vi "UI Set State.vi"(8 "error in (no error)":errorcluster, 10 "State Type":string, 11 "UI Refs":T1) -> (0 "error out":errorcluster, 3 "dup UI Refs":T1)   [LabVIEW 2015]
uses:
  controls/UI Data.ctl
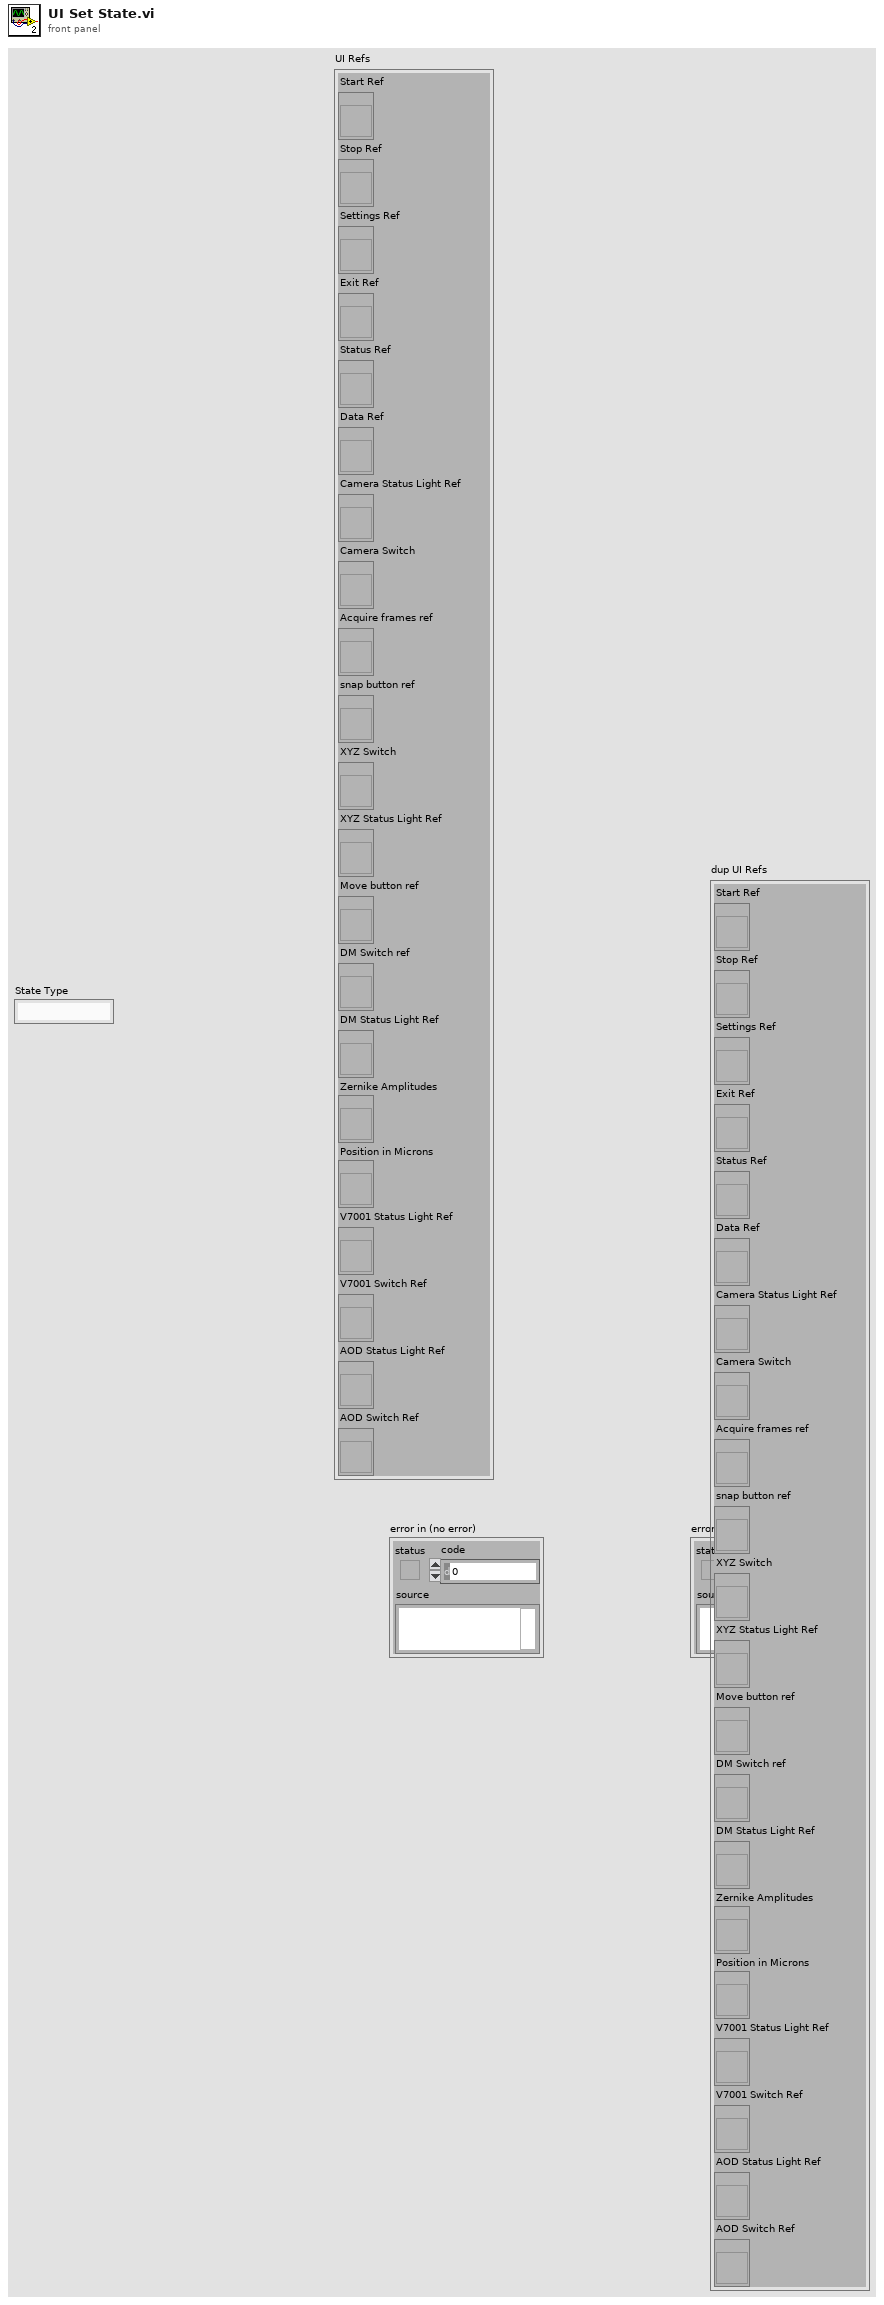
[diagram p1: front panel]
types:
  T1 = typedef "UI Data.ctl" = cluster{"Start Ref":refnum<vi>, "Stop Ref":refnum<vi>, "Settings Ref":refnum<vi>, "Exit Ref":refnum<vi>, "Status Ref":refnum<vi>, "Data Ref":refnum<vi>, "Camera Status Light Ref":refnum<vi>, "Camera Switch":refnum<vi>, "Acquire frames ref":refnum<vi>, "snap button ref":refnum<vi>, "XYZ Switch":refnum<vi>, "XYZ Status Light Ref":refnum<vi>, "Move button ref":refnum<vi>, "DM Switch ref":refnum<vi>, "DM Status Light Ref":refnum<vi>, "Zernike Amplitudes":refnum<vi>, "Position in Microns":refnum<vi>, "V7001 Status Light Ref":refnum<vi>, "V7001 Switch Ref":refnum<vi>, "AOD Status Light Ref":refnum<vi>, "AOD Switch Ref":refnum<vi>}
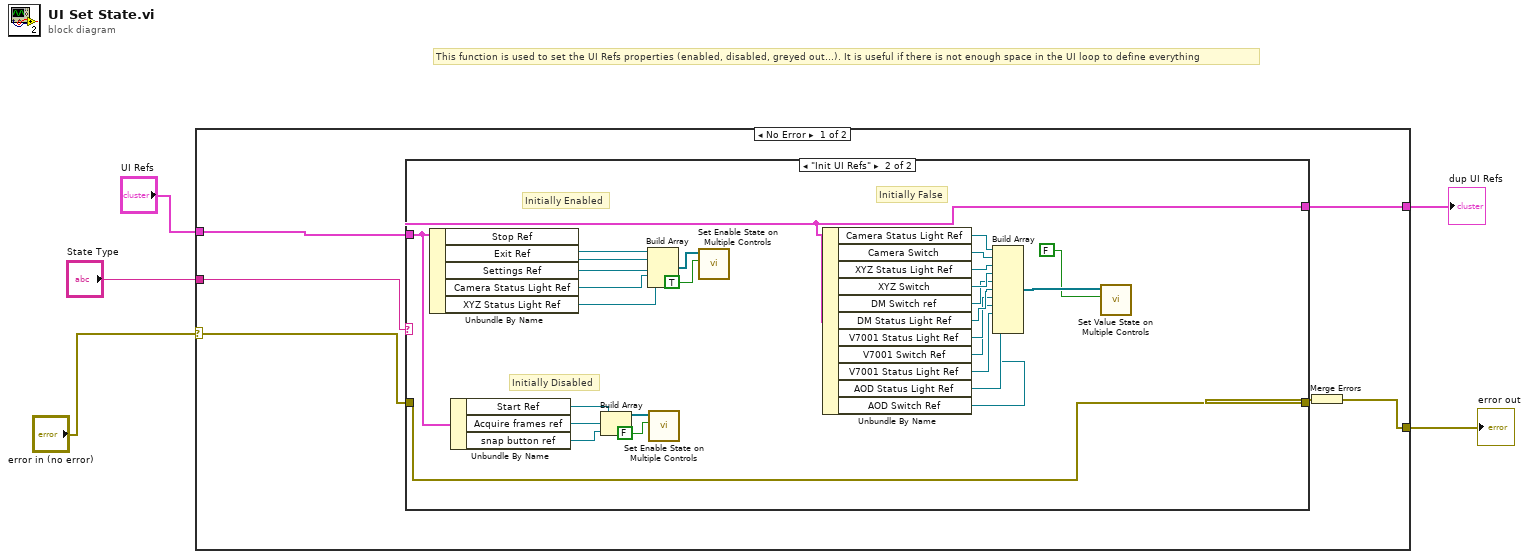
[diagram p0: block diagram]
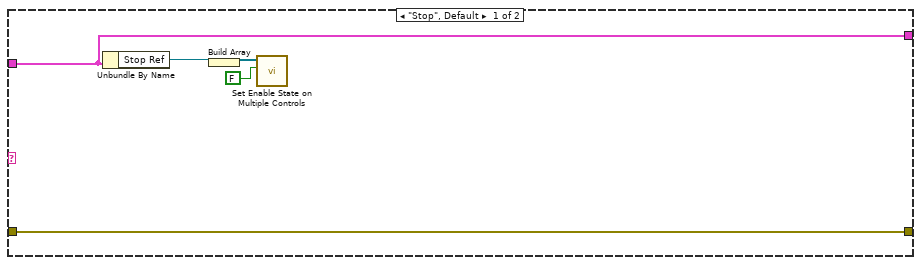
[diagram p2: hidden frame]
diagram:
  # "This function is used to set the UI Refs properties (enabled, disabled, greyed out...). It is useful if there is not enough space in the UI loop to define everything"
  n1 = case shown="No Error" "error in (no error)" {
    selector: "error in (no error)" -> [w7 w45]
    tunnel: [w10 w45] -> w4
    tunnel: "UI Refs" -> [w11 w44]
    tunnel: "State Type" -> [w8 _]
    tunnel: [w6 w44] -> w1
    frame No Error {
      n2 = case shown="\"Init UI Refs\"" w8 {
        tunnel: w11 -> [w12 w33]
        tunnel: [w16 w24] -> w9
        tunnel: w7 -> [w16 w24]
        tunnel: [w12 w33] -> w6
        frame "Stop", Default {
          n3 = Unbundle By Name(w12) -> ("Stop Ref"=w13:refnum<vi>)
          n4 = Build Array(w13) -> (w15:refnum<vi>[])
          n5 = call "Set Enable State on Multiple Controls.vi"("Enable?"=FALSE, "Controls"=w15) -> ()  [unwired: 10 in]
        }
        frame "Init UI Refs" {
          # "Initially False"
          # "Initially Disabled"
          # "Initially Enabled"
          n6 = Unbundle By Name(w33) -> ("Stop Ref"=w43:refnum<vi>, "Exit Ref"=w42:refnum<vi>, "Settings Ref"=w41:refnum<vi>, "Camera Status Light Ref"=w38:refnum<vi>, "XYZ Status Light Ref"=w31:refnum<vi>)
          n7 = Unbundle By Name(w33) -> ("Start Ref"=w35:refnum<vi>, "Acquire frames ref"=w34:refnum<vi>, "snap button ref"=w32:refnum<vi>)
          n8 = Build Array(w35, w34, w32) -> (w37:refnum<vi>[])
          n9 = Build Array(w43, w42, w41, w38, w31) -> (w39:refnum<vi>[])
          n10 = call "Set Enable State on Multiple Controls.vi"("Enable?"=FALSE, "Controls"=w37) -> ()  [unwired: 10 in]
          n11 = call "Set Enable State on Multiple Controls.vi"("Enable?"=TRUE, "Controls"=w39) -> ()  [unwired: 10 in]
          n12 = Unbundle By Name(w33) -> ("Camera Status Light Ref"=w30:refnum<vi>, "Camera Switch"=w29:refnum<vi>, "XYZ Status Light Ref"=w28:refnum<vi>, "XYZ Switch"=w27:refnum<vi>, "DM Switch ref"=w23:refnum<vi>, "DM Status Light Ref"=w22:refnum<vi>, "V7001 Status Light Ref"=w21:refnum<vi>, "V7001 Switch Ref"=w20:refnum<vi>, "V7001 Status Light Ref"=w19:refnum<vi>, "AOD Status Light Ref"=w18:refnum<vi>, "AOD Switch Ref"=w17:refnum<vi>)
          n13 = Build Array(w30, w29, w28, w27, w23, w22, w21, w20, w19, w18, w17) -> (w26:refnum<vi>[])
          n14 = call "Set Value State on Multiple Controls.vi"("Value"=FALSE ("Enable?"), "Controls"=w26) -> ()  [unwired: 10 in]
        }
      }
      n15 = Merge Errors(w9) -> (w10:errorcluster)
    }
    frame Error {
    }
  }
  "error out" <- w4
  "dup UI Refs" <- w1
